vi "SerialConsole.vi"() -> ()   [LabVIEW 2012]
panel:
  in  "send":bool
  in  "send":string
  out "concatenated string":string="\r\n\r\nSoftware reset\r\n\r\nFlash driver init successful\r\nFlash device recognized\r\nFlash device 0 init successful\r\nFlash device 1 init successful\r\nBoot flash cannot be write enabled\r\n\r\nPress any key to stop auto-boot...\r\n 1\r 0\r\r\nauto-booting...\r\n\r\n\r\nboot device          : ffx\r\nunit number          : 0 \r\nprocessor number     : 0 \r\nhost name            : lvrt\r\nfile name            : /c/ni-rt/system/vxWorks\r\nflags (f)            : 0x8 \r\n\r\nAttaching to flash device...\r\nLoading /c/ni-rt/system/vxWorks...3560608\r\nStarting at 0x10000...\r\n\r\nDatalight FlashFX Tera v1.2.3 Build 1850EY\r\nVxWorks 6.3 Edition for ppc603 -- Compiled Dec  2 2011 at 16:50:23\r\nCopyright (c) 1993-2010 Datalight, Inc.  All Rights Reserved Worldwide.\r\nReliance File System Driver\r\nDatalight Reliance v3.2.2 Build 1376BV\r\nVxWorks Edition for ppc603\r\nCopyright (c) 2003-2008 Datalight, Inc.  All Rights Reserved Worldwide.\r\n\r\nAdding 8864 symbols for standalone.\r\n\r\n-> * Loading vxfpsup.out: vxfpsup\r\nlvusEngine: PPC603 CPU detected...\r\nCPU tick frequency: 49.498875 MHz [Using: 1000 MHz]\r\n\r\nVxWorks kernel image\r\nBuild time: Dec  2 2011, 16:51:21\r\n\r\nLabVIEW Real-Time Executive\r\nBuild Time: Dec  4 2011 15:56:37\r\n(C) Copyright 2002-2011 National Instruments Corporation\r\n\r\nMAX system identification name: NI-sbRIO9636-0174E7E0\r\nInitializing network... \r\nDevice 1 - MAC addr: 00:80:2F:14:1B:42 - 169.254.66.100 /16 (primary - auto)\r\n* Loading nimdnsResponder.out: nimdnsResponder\r\nStarting mDNSResponder task tMDNS.\r\n* Loading nirtdm.out: nirtdm\r\n\r\nLoading LVRT...\r\n* Loading nirtdm.out: nirtdm\r\n* Loading nimdnsResponder.out: nimdnsResponder\r\n* Loading vxfpsup.out: vxfpsup\r\n* Loading tsengine.out: tsengine\r\n* Loading nisvcloc.out: nisvcloc\r\n* Loading RTWebServer.out: RTWebServer\r\nSystem Web Server started\r\n* Loading niDiscSvc.out: niDiscSvc\r\n* Loading nisysrpc.out: nisysrpc\r\n* Loading NiRioRpc.out: NiRioRpc\r\n* Loading nidp_target_end.out: nidp_target_end\r\nNI-RIO Server 4.1 started successfully.\r\nNI Scan Engine initialized.\r\n* Loading niorbs.out: niorbs\r\n* Loading niserial.out: niserial\r\n* Loading NiViSrvr.out: NiViSrvr\r\n* Loading sysstatepublisher.out: sysstatepublisher\r\n\r\nWelcome to LabVIEW Real-Time 11.0.1\r\n\r\nNI-VISA Server 5.1 started successfully.\r\n"
  in  "stop":bool
  # "192.168.0.5"
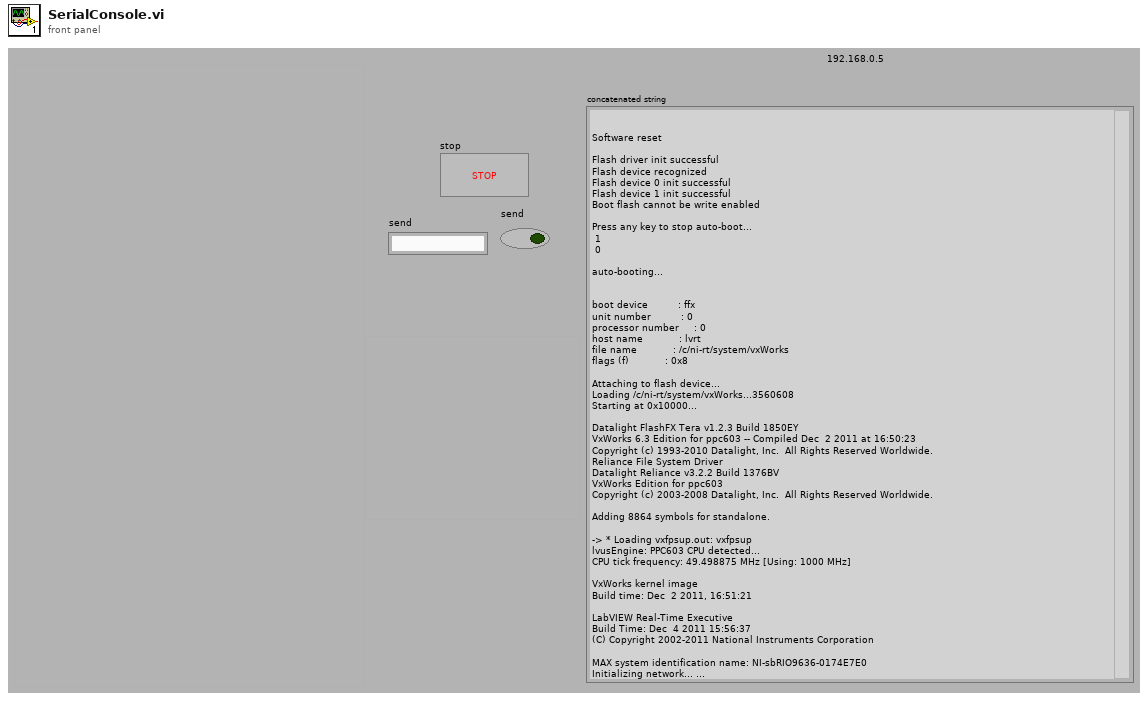
[diagram p1: front panel]
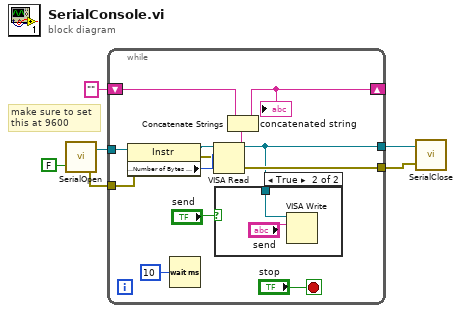
[diagram p0: block diagram]
diagram:
  # "make sure to set\nthis at 9600"
  n1 = call <userlib>:"SerialOpen.vi"("Check for Monitor"=FALSE) -> ("error out"=w4:errorcluster, "VISA resource name out"=w5:refnum<visa-resource-name>)  [unwired: 1 in]
  n2 = while {
    shift-right: [w18] -> _
    shift-left: "" -> [w19]
    tunnel: w5 -> [w17]
    tunnel: w4 -> [w16]
    tunnel: [w9] -> w3
    tunnel: [w11] -> w2
    stop <- "stop" stop-if-true
    n3 = property class="Instr"(reference=w17, error in=w16) -> (reference out=w15:refnum<visa-resource-name>, error out=w13:errorcluster, "Serial Settings:Number of Bytes at Serial Port"=w14:u32)
    n4 = Wait (ms)(milliseconds to wait=u32 10) -> ()  [unwired: 1 out]
    n5 = VISA Read(VISA resource name=w15, byte count=w14, error in (no error)=w13) -> (VISA resource name out=w9:refnum<visa-resource-name>, read buffer=w12:string, error out=w11:errorcluster)  [unwired: 1 out]
    n6 = case shown="True" "send" {
      tunnel: w9 -> [_ w21]
      frame False {
      }
      frame True {
        n7 = VISA Write(VISA resource name=w21, write buffer="send") -> ()  [unwired: 1 in, 3 out]
      }
    }
    n8 = Concatenate Strings(w19, w12) -> (w18:string)
    "concatenated string" <- w18
  }
  n9 = call <userlib>:"SerialClose.vi"("error in"=w2, "Serial Port"=w3) -> ()  [unwired: 2 in]
